vi "Combine Operation.vi"(5 "initialize entry (F)":bool, 6 "chip select  (1st chip)":enum16{"1st chip", "2nd chip"}(ring), 7 "function set (F)":bool, 8 "error in (no error)":errorcluster, 9 "cmd/data":u8 format="%.0x", 10 "RS":bool, 11 "R/W":bool) -> (0 "error out":errorcluster, 2 "output":u32 format="%.0x")   [LabVIEW 2017, in "HD44780.lvclass"]
uses:
  HD44780.lvclass
  Common/HD44780 Common.lvlib
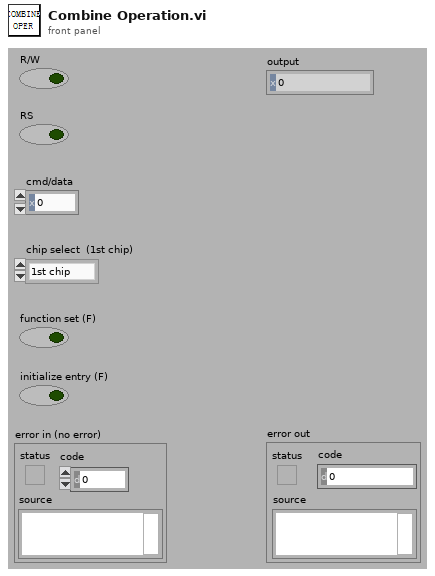
[diagram p1: front panel]
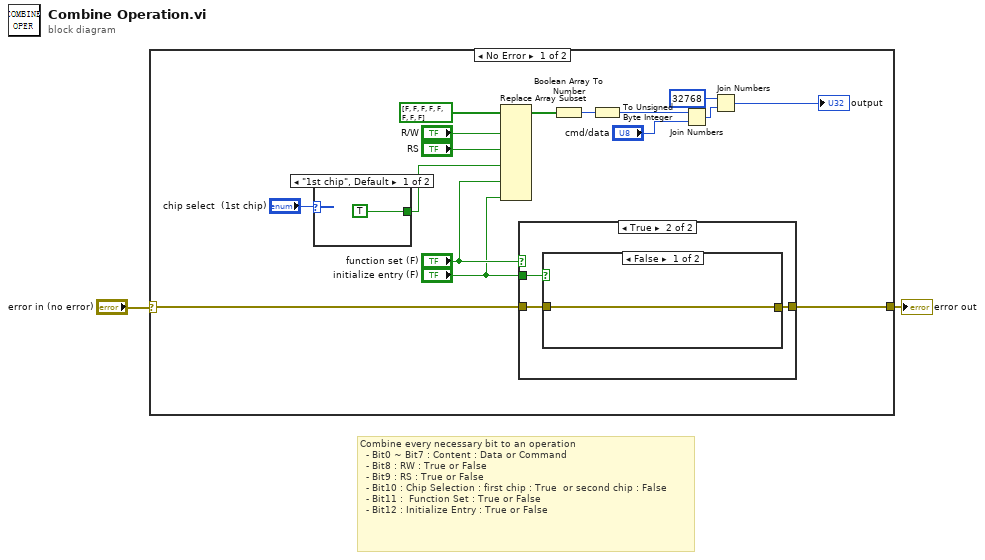
[diagram p0: block diagram]
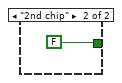
[diagram p2: hidden frame]
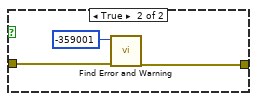
[diagram p4: hidden frame]
diagram:
  # "Combine every necessary bit to an operation\n  - Bit0 ~ Bit7 : Content : Data or Command\n  - Bit8 : RW : True or False\n  - Bit9 : RS : True or False\n  - Bit10 : Chip Selection : first chip : True  or second chip : False\n  - Bit11 :  Function Set : True or False\n  - Bit12 : Initialize Entry : True or False"
  n1 = case shown="No Error" "error in (no error)" {
    selector: "error in (no error)" -> [w10 w29]
    tunnel: [w11 w29] -> w1
    frame No Error {
      n2 = case shown="\"1st chip\", Default" "chip select  (1st chip)" {
        tunnel: [TRUE FALSE] -> w5
        frame "1st chip", Default {
        }
        frame "2nd chip" {
        }
      }
      n3 = Replace Array Subset(array=bool[] [FALSE, FALSE, FALSE, FALSE, FALSE, FALSE, FALSE, FALSE] ("initialized array"), new element #1="R/W", new element #2="RS", new element #3=w5, new element #4="function set (F)", new element #5="initialize entry (F)") -> (w8:bool[])  [unwired: 5 in]
      n4 = case shown="True" "function set (F)" {
        tunnel: "initialize entry (F)" -> [_ w24]
        tunnel: [w21 w23] -> w11
        tunnel: w10 -> [w21 w22]
        frame False {
        }
        frame True {
          n5 = case shown="False" w24 {
            tunnel: [w25 w28] -> w23
            tunnel: w22 -> [w25 w26]
            frame False {
            }
            frame True {
              n6 = call "Find Error and Warning.vi"("error in (no error)"=w26, "error code"=-359001) -> ("error out"=w28:errorcluster)  [unwired: 9 in]
            }
          }
        }
      }
      n7 = Boolean Array To Number(Boolean array=w8) -> (number=w16:u32)
      n8 = To Unsigned Byte Integer(number=w16) -> (unsigned 8bit integer=w15:u8)
      n9 = Join Numbers(hi=w15, lo="cmd/data") -> ((hi.lo)=w14:u16)
      n10 = Join Numbers(hi=u16 32768, lo=w14) -> ((hi.lo)=→"output":u32)
    }
    frame Error {
    }
  }
  "error out" <- w1
